vi "Init Device.vi"(7 "Layout Ref":refnum<vi>, 8 "error in (no error)":errorcluster, 10 "Chan# Array":i32[](array[numeric]), 11 "Advanced_DMD in":refnum<class "Advanced_DMD.lvclass">) -> (0 "error out":errorcluster, 3 "Advanced_DMD out":refnum<class "Advanced_DMD.lvclass">)   [LabVIEW 2013, in "Advanced_DMD.lvclass"]
doc: "Initialize the correct columns and their default appearance.\nUse the front panel to change default appearance of the device in the Add/Manage devices.\n\nOpen a specific device implementation for details."
uses:
  Advanced_DMD.lvclass
  TypeDefs/ColumnAppearCluster.ctl
  ColumnVIs/MenuDisableCol/MenuDisableCol.lvclass
  ColumnVIs/MenuDisableCol/MenuItemDisables.ctl
  ColumnVIs/SingleValCol/SingleValCol.lvclass
  ColumnVIs/SingleValMenuCol/SingleValMenuCol.lvclass
  ColumnVIs/Column/Column.lvclass
panel:
  in  "MenuItemList":string[](array[string])=["Static Image", "Pattern Sequence"]
  in  "Display Mode Appearance":T1={"Column Name"="Disp Mode", "Width"=30, "Bkgd"=[16448250], "Text"=[0]}
  in  "Program Mode Appearance":T1={"Column Name"="Program Mode", "Width"=30, "Bkgd"=[16448250], "Text"=[0]}
  in  "MenuItemList 2":string[](array[string])=["Always Upload", "Upload Changes Only"]
  in  "ArgumentColAppear":T1={"Column Name"="", "Width"=30, "Bkgd"=[16448250], "Text"=[0]}
  in  "MenuColAppear":T1={"Column Name"="", "Width"=30, "Bkgd"=[16448250], "Text"=[0]}
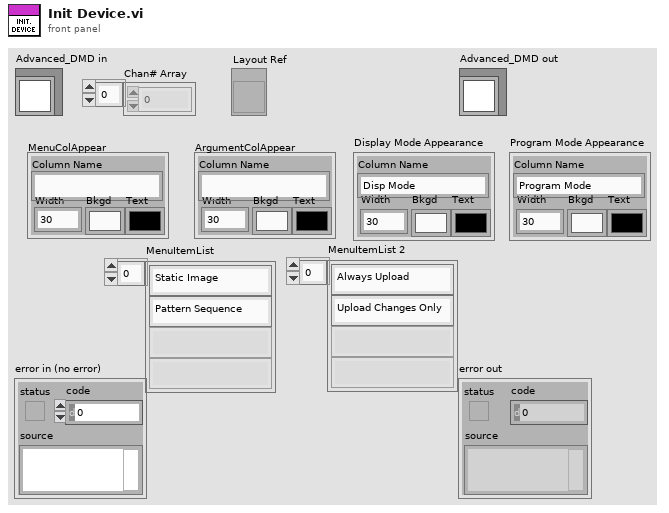
[diagram p1: front panel]
types:
  T1 = typedef "ColumnAppearCluster.ctl" = cluster{"Column Name":string, "Width":u32, "Bkgd":u32[], "Text":u32[]}
  T2 = typedef "MenuItemDisables.ctl" = cluster{"MenuEntry":string, "DisableColumns":i32[]}
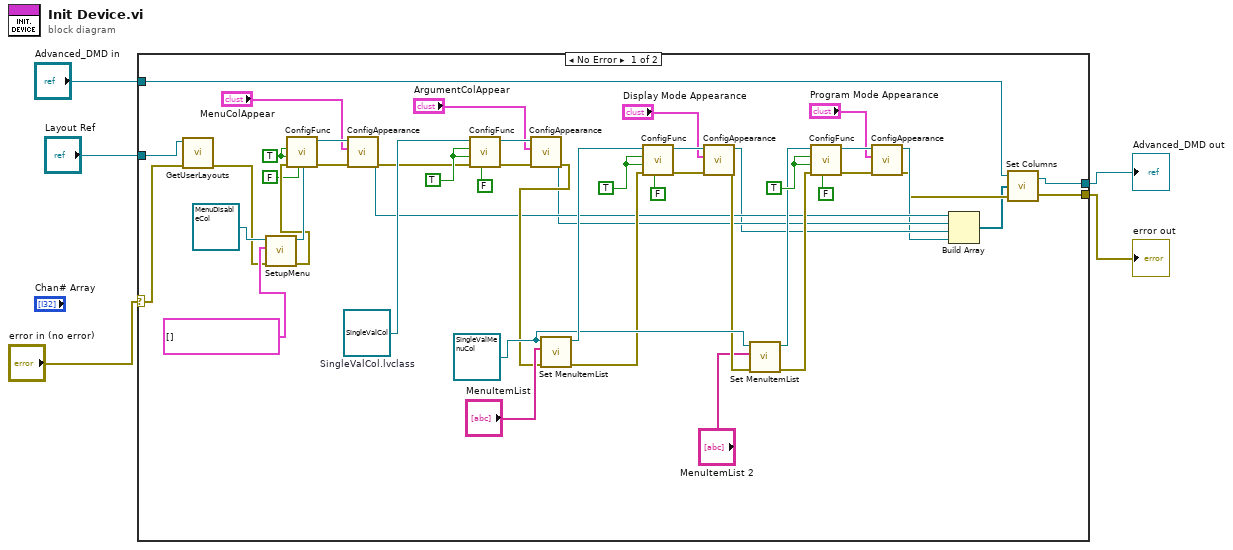
[diagram p0: block diagram]
diagram:
  n1 = case shown="No Error" "error in (no error)" {
    selector: "error in (no error)" -> [w51 w53]
    tunnel: "Layout Ref" -> [w52 _]
    tunnel: "Advanced_DMD in" -> [w8 w54]
    tunnel: [w7 w54] -> w2
    tunnel: [w6 w53] -> w1
    frame No Error {
      w28 = TRUE ("Disableable? (True)")
      w32 = TRUE ("Disableable? (True)")
      w21 = refnum<class "SingleValMenuCol.lvclass"> refnum ("SingleValMenuCol.lvclass")
      w38 = TRUE ("Disableable? (True)")
      w40 = refnum<class "SingleValCol.lvclass"> refnum  # SingleValCol.lvclass
      w44 = TRUE ("isVariable? (True)")
      n2 = call "GetUserLayouts.vi"("error in (no error)"=w51, "Layout Ring Refnum"=w52) -> ("error out"=w47:errorcluster)  [unwired: 5 in, 4 out]
      n3 = call-dynamic "SetupMenu.vi"("error in (no error)"=w47, "MenuItemDisablesList"=T2[] [], "MenuDisableCol in"=refnum<class "MenuDisableCol.lvclass"> refnum ("MenuDisableCol.lvclass")) -> ("error out"=w46:errorcluster, "MenuDisableCol out"=w48:refnum<class "MenuDisableCol.lvclass">)  [unwired: 7 in]
      n4 = call "ConfigFunc.vi"("isRampable? (True"=FALSE, "error in (no error)"=w46, "isVariable? (True)"=w44, "Disableable? (True)"=w44, "Column in"=w48) -> ("error out"=w45:errorcluster, "Column out"=w42:refnum<class "MenuDisableCol.lvclass">)  [unwired: 5 in]
      n5 = call "ConfigAppearance.vi"("error in (no error)"=w45, "Column Appearance"="MenuColAppear", "Column in"=w42) -> ("error out"=w36:errorcluster, "Column out"=w14:refnum<class "MenuDisableCol.lvclass">)  [unwired: 7 in]
      n6 = call "ConfigFunc.vi"("isRampable? (True"=FALSE, "error in (no error)"=w36, "isVariable? (True)"=w38, "Disableable? (True)"=w38, "Column in"=w40) -> ("error out"=w35:errorcluster, "Column out"=w39:refnum<class "SingleValCol.lvclass">)  [unwired: 5 in]
      n7 = call "ConfigAppearance.vi"("error in (no error)"=w35, "Column Appearance"="ArgumentColAppear", "Column in"=w39) -> ("error out"=w19:errorcluster, "Column out"=w13:refnum<class "SingleValCol.lvclass">)  [unwired: 7 in]
      n8 = call-dynamic "Set MenuItemList.vi"("error in (no error)"=w19, "MenuItemList"="MenuItemList", "MenuCol in"=w21) -> ("error out"=w18:errorcluster, "MenuCol out"=w24:refnum<class "SingleValMenuCol.lvclass">)  [unwired: 7 in]
      n9 = call "ConfigFunc.vi"("isRampable? (True"=FALSE, "error in (no error)"=w18, "isVariable? (True)"=w32, "Disableable? (True)"=w32, "Column in"=w24) -> ("error out"=w30:errorcluster, "Column out"=w33:refnum<class "SingleValMenuCol.lvclass">)  [unwired: 5 in]
      n10 = call "ConfigAppearance.vi"("error in (no error)"=w30, "Column Appearance"="Display Mode Appearance", "Column in"=w33) -> ("error out"=w17:errorcluster, "Column out"=w12:refnum<class "SingleValMenuCol.lvclass">)  [unwired: 7 in]
      n11 = call-dynamic "Set MenuItemList.vi"("error in (no error)"=w17, "MenuItemList"="MenuItemList 2", "MenuCol in"=w21) -> ("error out"=w16:errorcluster, "MenuCol out"=w20:refnum<class "SingleValMenuCol.lvclass">)  [unwired: 7 in]
      n12 = call "ConfigFunc.vi"("isRampable? (True"=FALSE, "error in (no error)"=w16, "isVariable? (True)"=w28, "Disableable? (True)"=w28, "Column in"=w20) -> ("error out"=w26:errorcluster, "Column out"=w29:refnum<class "SingleValMenuCol.lvclass">)  [unwired: 5 in]
      n13 = call "ConfigAppearance.vi"("error in (no error)"=w26, "Column Appearance"="Program Mode Appearance", "Column in"=w29) -> ("error out"=w10:errorcluster, "Column out"=w11:refnum<class "SingleValMenuCol.lvclass">)  [unwired: 7 in]
      n14 = Build Array(w14, w13, w12, w11) -> (w9:refnum<class "Column.lvclass">[])
      n15 = call-dynamic "Set Columns.vi"("error in (no error)"=w10, "Columns"=w9, "Device in"=w8) -> ("error out"=w6:errorcluster, "Device out"=w7:refnum<class "Advanced_DMD.lvclass">)  [unwired: 1 in]
    }
    frame Error {
    }
  }
  "error out" <- w1
  "Advanced_DMD out" <- w2
